vi "Static Read.vi"(8 "error in (no error)":errorcluster, 11 "Abs_Boolean in":refnum<class "Abs_Boolean.lvclass">) -> (0 "error out":errorcluster, 2 "Boolean":bool, 3 "Abs_Boolean out":refnum<class "Abs_Boolean.lvclass">)   [LabVIEW 2021, in "Abs_Boolean.lvclass"]
uses:
  Abs_Boolean.lvclass
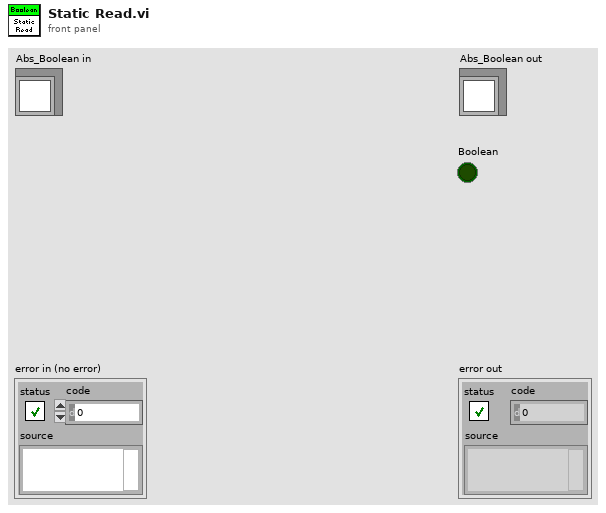
[diagram p1: front panel]
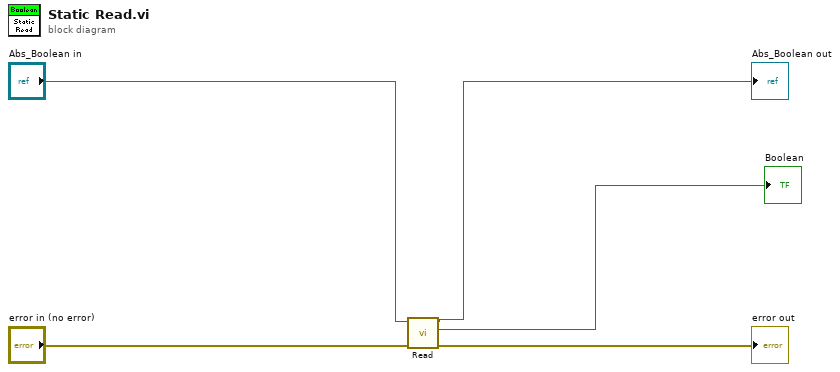
[diagram p0: block diagram]
diagram:
  n1 = call-dynamic "Read.vi"("error in (no error)"="error in (no error)", "Boolean in"="Abs_Boolean in") -> ("error out"=→"error out":errorcluster, "Boolean"=→"Boolean":bool, "Boolean out"=→"Abs_Boolean out":refnum<class "Abs_Boolean.lvclass">)  [unwired: 7 in]
